vi "DHE_ChangeRawBpp.vi"(8 "error in (no error)":errorcluster, 10 "bpp":i32, 11 "fd":i32) -> (0 "error out":errorcluster, 3 "fd out":i32)   [LabVIEW 2016]
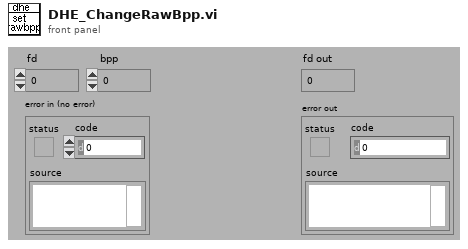
[diagram p1: front panel]
types:
  T1 = typedef "GEOM_CorrectedFPA.ctl" = cluster{"readmode":string, "amplifiers":cluster{"number":i32, "xstart":i32, "ystart":i32}[], "totxsize":i32, "totysize":i32, "maxxdim":i32, "maxydim":i32, "numxamps":i32, "numyamps":i32, "totxdata":i32, "totydata":i32, "xdataamp":i32, "ydataamp":i32, "totpixels":i32}
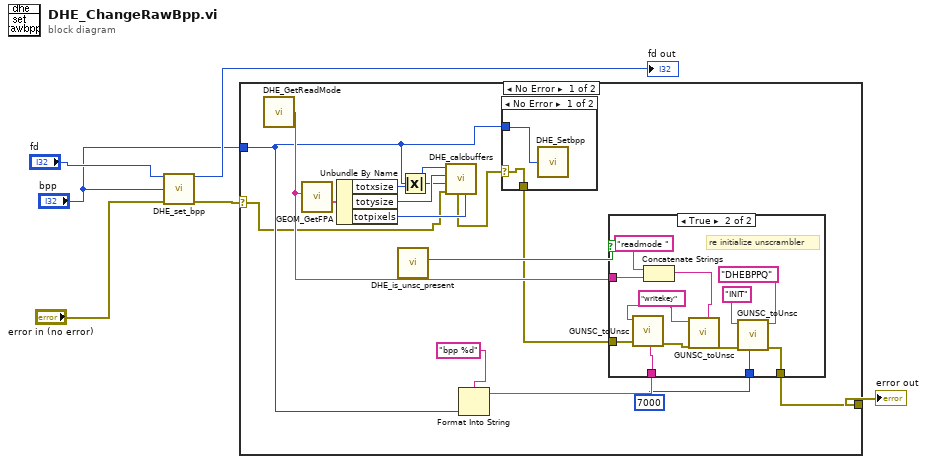
[diagram p0: block diagram]
diagram:
  n1 = call "DHE_set_bpp.vi"("fd"="fd", "bpp"="bpp", "error in (no error)"="error in (no error)") -> ("fd out"=→"fd out":i32, "error out"=w6:errorcluster)  [unwired: 11 out]
  n2 = case shown="No Error" w6 {
    selector: w6 -> [w11 w38]
    tunnel: "bpp" -> [w12 _]
    tunnel: [w13 w38] -> w1
    frame No Error {
      n3 = call "DHE_GetReadMode.vi"() -> ("DHE_ReadMode"=w19:string)  [unwired: 9 out]
      n4 = call "GEOM_GetFPA.vi"("readmode"=w19) -> ("CorrectedFPACoord"=w21:T1)  [unwired: 2 in, 8 out]
      n5 = Unbundle By Name(w21) -> ("totxsize"=w15:i32, "totysize"=w14:i32, "totpixels"=w20:i32)
      n6 = call "DHE_is_unsc_present.vi"() -> ("value"=w18:bool)  [unwired: 1 in, 10 out]
      n7 = Absolute Value(x=w12) -> (abs(x)=w8:i32)
      n8 = call "DHE_calcbuffers.vi"("totpixelsin"=w20, "error in (no error)"=w11, "bpp"=w8, "nrows"=w14, "ncols"=w15) -> ("error out"=w10:errorcluster)  [unwired: 1 in, 5 out]
      n9 = Format Into String(format string="bpp %d", w12) -> (resulting string=w17:string)  [unwired: 2 in, 1 out]
      n10 = case shown="No Error" w10 {
        selector: w10 -> [w22 w24]
        tunnel: w12 -> [w23 _]
        tunnel: [w22 w24] -> w9
        frame No Error {
          n11 = call "DHE_Setbpp.vi"("DHE_bpp"=w23) -> ()  [unwired: 9 out]
        }
        frame Error {
        }
      }
      n12 = case shown="True" w18 {
        tunnel: [w25 w32] -> w13
        tunnel: w9 -> [w25 w31]
        tunnel: 7000 ("ms timeout (-1)") -> [_ w29]
        tunnel: w19 -> [_ w27]
        tunnel: w17 -> [_ w26]
        frame False {
        }
        frame True {
          w28 = "writekey" ("command")
          # "re initialize unscrambler"
          n13 = call "GUNSC_toUnsc.vi"("key"=w26, "error in (no error)"=w31, "command"=w28) -> ("error out"=w30:errorcluster)  [unwired: 6 in, 2 out]
          n14 = Concatenate Strings("readmode " ("string"), w27) -> (w35:string)
          n15 = call "GUNSC_toUnsc.vi"("key"=w35, "error in (no error)"=w30, "command"=w28) -> ("error out"=w37:errorcluster)  [unwired: 6 in, 2 out]
          n16 = call "GUNSC_toUnsc.vi"("responseQ"="DHEBPPQ", "bpp"=w29, "error in (no error)"=w37, "command"="INIT") -> ("error out"=w32:errorcluster)  [unwired: 5 in, 2 out]
        }
      }
    }
    frame Error {
    }
  }
  "error out" <- w1
